vi "rs3_MemCopyRGB_IR2.vi"(0 "Zimage pointer":u64, 5 "RGB  X, width":i32, 7 "RGB Y, height":i32, 9 "Color format":enum16{"Monochrome", "RGB internal (RGB)"}(ring), 11 "error in (no error)":errorcluster) -> (4 "Output Array":u8[](array[numeric]), 10 "Length":i32=10, 15 "error out":errorcluster)   [LabVIEW 2019, in "libRealSense3.lvlib"]
doc: "Use this after a getZimage function call, to copy the memory pointed to, into an 2D array in LabVIEW."
uses:
  libRealSense3.lvlib
panel:
  # "RS3_Mem Copy_RGB/IR"
  # "(C) Intel Corp.,  AGJ"
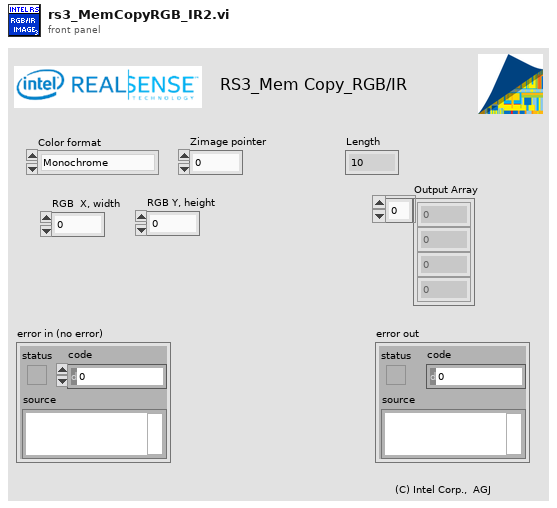
[diagram p1: front panel]
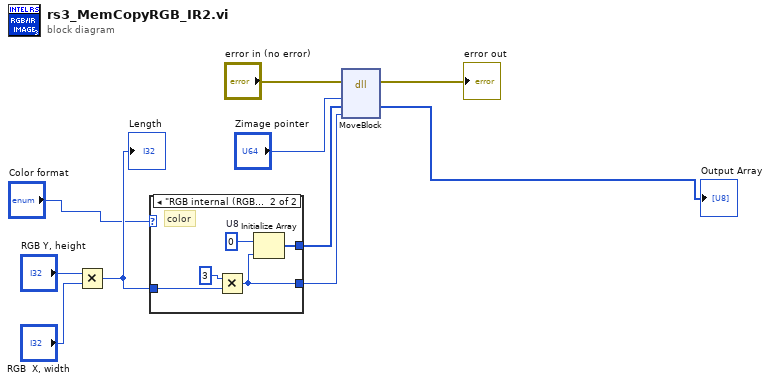
[diagram p0: block diagram]
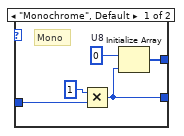
[diagram p2: hidden frame]
diagram:
  n1 = Multiply(x="RGB Y, height", y="RGB  X, width") -> (x*y=w6:i32)
  "Length" <- w6
  n2 = case shown="\"RGB internal (RGB)\"" "Color format" {
    tunnel: [w14 w17] -> w7
    tunnel: w6 -> [w13 w18]
    tunnel: [w12 w16] -> w5
    frame "Monochrome", Default {
      w15 = u8 0  # U8
      # "Mono"
      n3 = Multiply(x=1 ("# of bytes/number"), y=w13) -> (x*y=w12:i32)
      n4 = Initialize Array(w15, w12) -> (w14:u8[])
    }
    frame "RGB internal (RGB)" {
      w20 = u8 0  # U8
      # "color"
      n5 = Multiply(x=3 ("# of bytes/number"), y=w18) -> (x*y=w16:i32)
      n6 = Initialize Array(w20, w16) -> (w17:u8[])
    }
  }
  n7 = dll-call lib="LabVIEW" fn="MoveBlock"(error in="error in (no error)", "Address(Pointer)"="Zimage pointer", "Destination"=w7, "Size"=w5) -> (error out=→"error out":errorcluster, "Destination"=→"Output Array":u8[])  [unwired: 5 in, 1 out]
